vi "Name.vi"(8 "error in":errorcluster, 11 "NonOOPlayer in":refnum<class "NonOOPlayer.lvclass">) -> (0 "error out":errorcluster, 2 "Name":string, 3 "NonOOPlayer out":refnum<class "NonOOPlayer.lvclass">)   [LabVIEW 2020, in "NonOOPlayer.lvclass"]
uses:
  NonOOPlayer.lvclass
  NonOOPlayer.lvlib
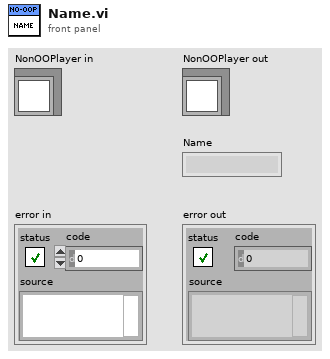
[diagram p1: front panel]
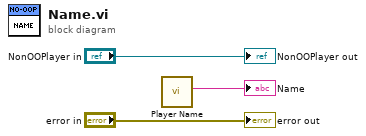
[diagram p0: block diagram]
diagram:
  n1 = call "Player Name.vi"() -> ("Name"=→"Name":string)  [unwired: 11 in]
  "error out" <- "error in"
  "NonOOPlayer out" <- "NonOOPlayer in"
